vi "Script Add Custom Error -- Library.vi"(2 "Selection Type":T1, 4 "Selection Owning Folder":path, 5 "Error Code":i32, 6 "Error Description":string, 7 "Error Name":string="TESTING.vi", 8 "error in":errorcluster, 9 "Error Arguments Window Ref":refnum<vi>, 10 "Project Reference":refnum<vi>, 11 "Library Ref":refnum<vi>) -> (0 "error out":errorcluster, 3 "Error VI Path":path)   [LabVIEW 2020, in "ConstantErrorsMaker.lvlib"]
uses:
  ConstantErrorsMaker.lvlib
  Selection Type--enum.ctl
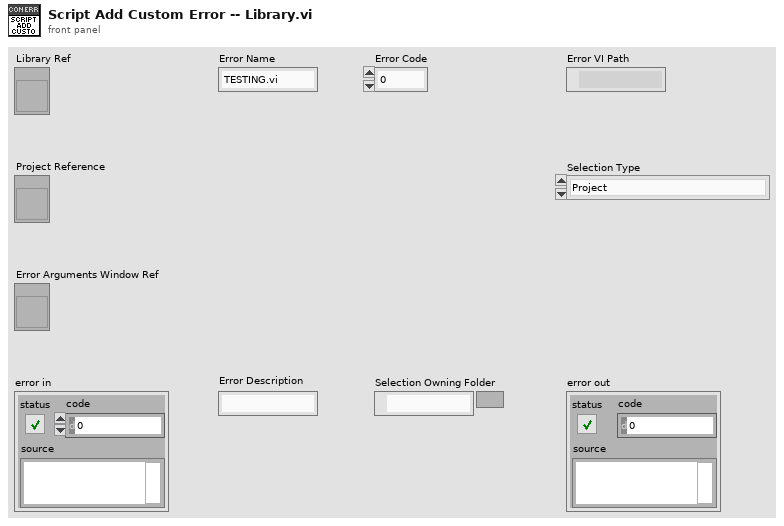
[diagram p1: front panel]
types:
  T1 = typedef "ConstantErrorsMaker.lvlib/Selection Type--enum.ctl" = enum16{"Project", "Library", "Class", "DQMH Singleton", "DQMH Cloneable"}
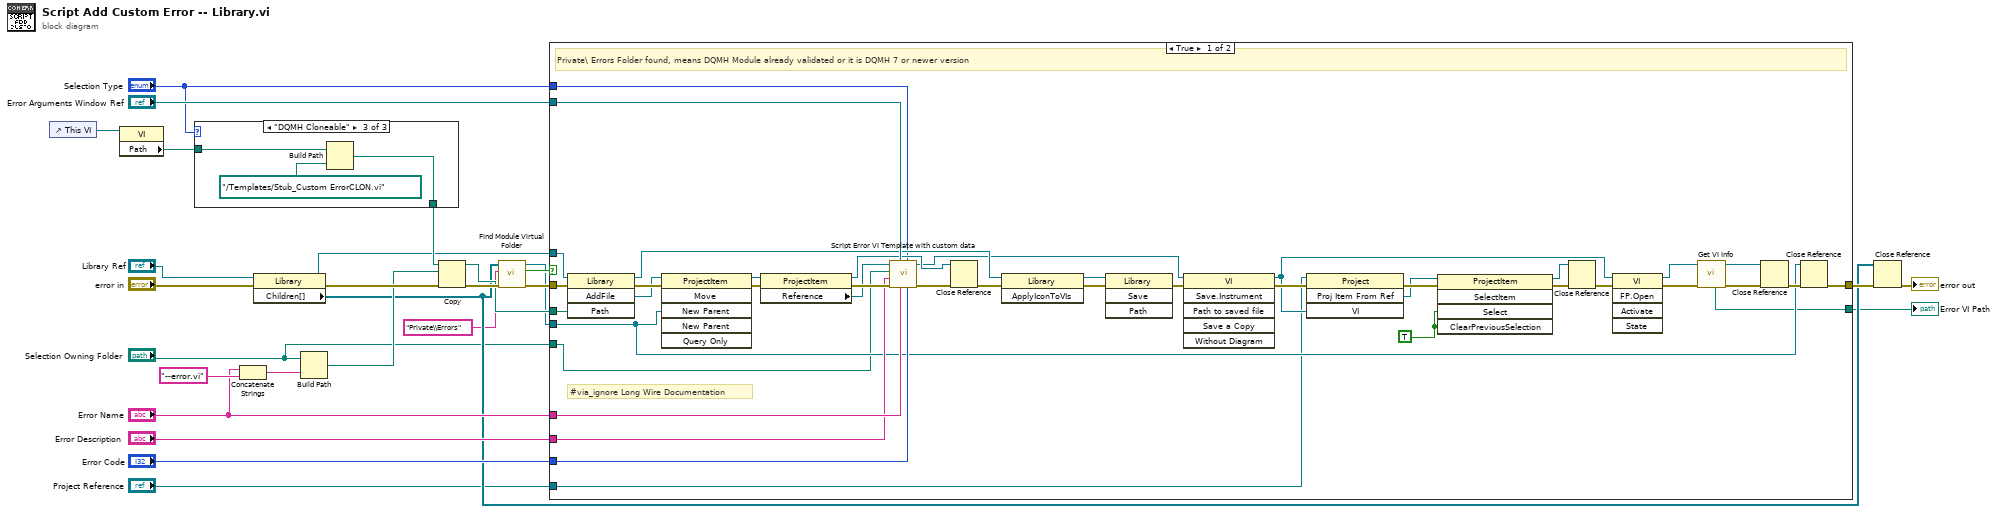
[diagram p0: block diagram]
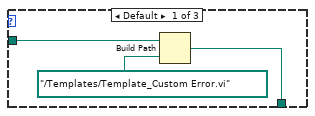
[diagram p2: hidden frame]
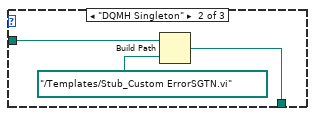
[diagram p3: hidden frame]
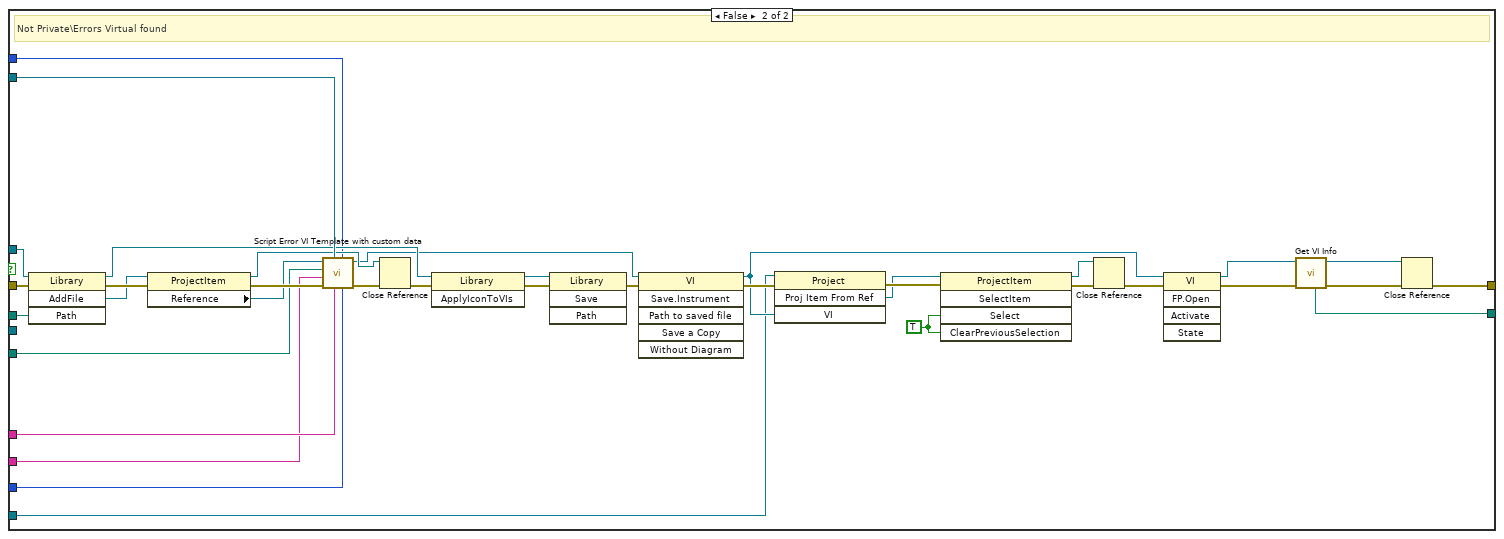
[diagram p4: hidden frame]
diagram:
  n1 = control-ref of="This VI"() -> (w19:refnum<vi>)
  n2 = property class="VI"(reference=w19) -> ("Path"=w18:path)  [unwired: 1 in, 2 out]
  n3 = case shown="\"DQMH Cloneable\"" "Selection Type" {
    tunnel: w18 -> [w30 w33 w36]
    tunnel: [w28 w31 w34] -> w17
    frame Default {
      n4 = Build Path(base path=w30, name or relative path=path "../Templates/Template_Custom Error.vi") -> (appended path=w28:path)
    }
    frame "DQMH Singleton" {
      n5 = Build Path(base path=w33, name or relative path=path "../Templates/Stub_Custom ErrorSGTN.vi") -> (appended path=w31:path)
    }
    frame "DQMH Cloneable" {
      n6 = Build Path(base path=w36, name or relative path=path "../Templates/Stub_Custom ErrorCLON.vi") -> (appended path=w34:path)
    }
  }
  n7 = Concatenate Strings("Error Name", "--error.vi" ("input 1")) -> (w21:string)
  n8 = property class="Library"(reference="Library Ref", error in="error in") -> (reference out=w16:refnum<vi>, error out=w22:errorcluster, "Children[]"=w9:refnum<vi>[])
  n9 = Build Path(base path="Selection Owning Folder", name or relative path=w21) -> (appended path=w20:path)
  n10 = Copy(8:w22, 10:w20, 11:w17) -> (0:w23:errorcluster, 3:w14:path)  [unwired: 2 in, 1 out]
  n11 = call "Find Module Virtual Folder.vi"("error in"=w23, "Virtual Folder"="Private\\Errors", "Children"=w9) -> ("error out"=w24:errorcluster, "Found?"=w8:bool, "ProjectItem out"=w7:refnum<vi>)  [unwired: 6 in]
  n12 = case shown="True" w8 {
    tunnel: [w74 w107] -> w27
    tunnel: w16 -> [w59 w97]
    tunnel: w14 -> [w60 w98]
    tunnel: "Error Name" -> [w53 w92]
    tunnel: "Error Code" -> [w56 w95]
    tunnel: "Error Arguments Window Ref" -> [w55 w94]
    tunnel: "Error Description" -> [w49 w88]
    tunnel: w7 -> [w48 _]
    tunnel: w24 -> [w68 w101]
    tunnel: "Project Reference" -> [w46 w84]
    tunnel: [w39 w79] -> w3
    tunnel: "Selection Type" -> [w38 w78]
    tunnel: "Selection Owning Folder" -> [w37 w77]
    frame True {
      w43 = TRUE ("Select")
      # "#via_ignore Long Wire Documentation"
      # "Private\\ Errors Folder found, means DQMH Module already validated or it is DQMH 7 or newer version"
      n13 = invoke class="Library" method="AddFile"(reference=w59, error in=w68, "Path"=w60) -> (reference out=w52:refnum<vi>, error out=w75:errorcluster, "AddFile"=w58:refnum<vi>)  [unwired: 1 in, 1 out]
      n14 = invoke class="ProjectItem" method="Move"(reference=w58, error in=w75, "New Parent"=w48) -> (reference out=w57:refnum<vi>, error out=w76:errorcluster)  [unwired: 3 in, 4 out]
      n15 = property class="ProjectItem"(reference=w57, error in=w76) -> (reference out=w54:refnum<vi>, error out=w64:errorcluster, "Reference"=w45:refnum<vi>)
      n16 = call "Script Error VI Template with custom data.vi"("Error Code"=w56, "Selection Type"=w38, "Error Name"=w53, "Error Arguments Window Ref"=w55, "error in"=w64, "Error Description"=w49, "Library Path"=w37, "VI Ref Error in"=w45) -> ("error out"=w66:errorcluster, "Custom Error VI Ref"=w50:refnum<vi>)  [unwired: 2 in]
      n17 = Close Reference(reference=w54, error in (no error)=w66) -> (error out=w73:errorcluster)
      n18 = invoke class="Library" method="ApplyIconToVIs"(reference=w52, error in=w73) -> (reference out=w51:refnum<vi>, error out=w72:errorcluster)  [unwired: 1 in, 1 out]
      n19 = invoke class="Library" method="Save"(reference=w51, error in=w72) -> (error out=w71:errorcluster)  [unwired: 2 in, 3 out]
      n20 = invoke class="VI" method="Save.Instrument"(reference=w50, error in=w71) -> (reference out=w47:refnum<vi>, error out=w67:errorcluster)  [unwired: 4 in, 4 out]
      n21 = invoke class="Project" method="Proj Item From Ref"(reference=w46, error in=w67, "VI"=w47) -> (error out=w63:errorcluster, "ProjItemFromRef"=w44:refnum<vi>)  [unwired: 1 in, 2 out]
      n22 = invoke class="ProjectItem" method="SelectItem"(reference=w44, error in=w63, "Select"=w43, "ClearPreviousSelection"=w43) -> (reference out=w42:refnum<vi>, error out=w62:errorcluster)  [unwired: 1 in, 3 out]
      n23 = Close Reference(reference=w42, error in (no error)=w62) -> (error out=w65:errorcluster)
      n24 = invoke class="VI" method="FP.Open"(reference=w47, error in=w65) -> (reference out=w41:refnum<vi>, error out=w70:errorcluster)  [unwired: 3 in, 3 out]
      n25 = call "Get VI Info.vi"("error in"=w70, "VI in"=w41) -> ("error out"=w61:errorcluster, "VI out"=w40:refnum<vi>, "VI Path"=w39:path)  [unwired: 4 in, 3 out]
      n26 = Close Reference(reference=w40, error in (no error)=w61) -> (error out=w69:errorcluster)
      n27 = Close Reference(reference=w48, error in (no error)=w69) -> (error out=w74:errorcluster)
    }
    frame False {
      w86 = TRUE ("Select")
      # "Not Private\\Errors Virtual found"
      n28 = invoke class="Library" method="AddFile"(reference=w97, error in=w101, "Path"=w98) -> (reference out=w91:refnum<vi>, error out=w112:errorcluster, "AddFile"=w96:refnum<vi>)  [unwired: 1 in, 1 out]
      n29 = property class="ProjectItem"(reference=w96, error in=w112) -> (reference out=w93:refnum<vi>, error out=w100:errorcluster, "Reference"=w82:refnum<vi>)
      n30 = call "Script Error VI Template with custom data.vi"("Error Code"=w95, "Selection Type"=w78, "Error Name"=w92, "Error Arguments Window Ref"=w94, "error in"=w100, "Error Description"=w88, "Library Path"=w77, "VI Ref Error in"=w82) -> ("error out"=w103:errorcluster, "Custom Error VI Ref"=w89:refnum<vi>)  [unwired: 2 in]
      n31 = Close Reference(reference=w93, error in (no error)=w103) -> (error out=w111:errorcluster)
      n32 = invoke class="Library" method="ApplyIconToVIs"(reference=w91, error in=w111) -> (reference out=w90:refnum<vi>, error out=w110:errorcluster)  [unwired: 1 in, 1 out]
      n33 = invoke class="Library" method="Save"(reference=w90, error in=w110) -> (error out=w109:errorcluster)  [unwired: 2 in, 3 out]
      n34 = invoke class="VI" method="Save.Instrument"(reference=w89, error in=w109) -> (reference out=w85:refnum<vi>, error out=w105:errorcluster)  [unwired: 4 in, 4 out]
      n35 = invoke class="Project" method="Proj Item From Ref"(reference=w84, error in=w105, "VI"=w85) -> (error out=w106:errorcluster, "ProjItemFromRef"=w87:refnum<vi>)  [unwired: 1 in, 2 out]
      n36 = invoke class="ProjectItem" method="SelectItem"(reference=w87, error in=w106, "Select"=w86, "ClearPreviousSelection"=w86) -> (reference out=w83:refnum<vi>, error out=w104:errorcluster)  [unwired: 1 in, 3 out]
      n37 = Close Reference(reference=w83, error in (no error)=w104) -> (error out=w102:errorcluster)
      n38 = invoke class="VI" method="FP.Open"(reference=w85, error in=w102) -> (reference out=w81:refnum<vi>, error out=w108:errorcluster)  [unwired: 3 in, 3 out]
      n39 = call "Get VI Info.vi"("error in"=w108, "VI in"=w81) -> ("error out"=w99:errorcluster, "VI out"=w80:refnum<vi>, "VI Path"=w79:path)  [unwired: 4 in, 3 out]
      n40 = Close Reference(reference=w80, error in (no error)=w99) -> (error out=w107:errorcluster)
    }
  }
  "Error VI Path" <- w3
  n41 = Close Reference(reference=w9, error in (no error)=w27) -> (error out=→"error out":errorcluster)
